vi "Log File Creater.vi"(11 "FTP log file path":path) -> (0 "all condition error":errorcluster, 2 "File Refnum":refnum<file>, 3 "Created Path":path)   [LabVIEW 2012]
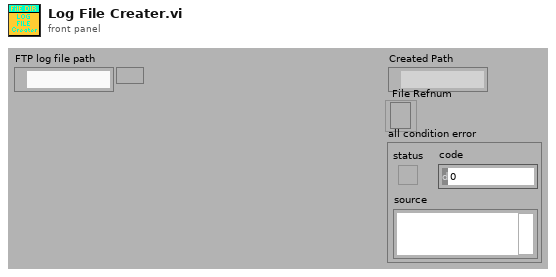
[diagram p1: front panel]
types:
  T1 = enum16{"open", "replace", "create", "open or create", "replace or create", "replace or create with confirmation"}
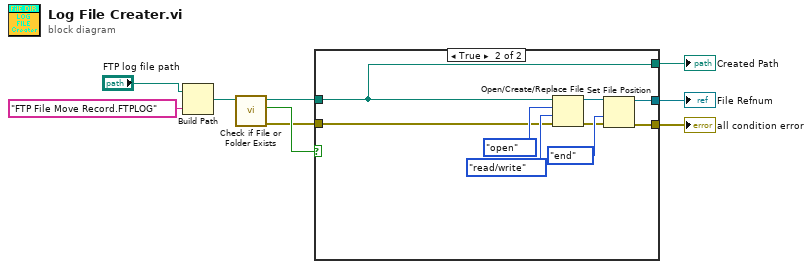
[diagram p0: block diagram]
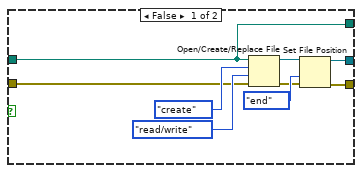
[diagram p2: hidden frame]
diagram:
  n1 = Build Path(base path="FTP log file path", name or relative path="FTP File Move Record.FTPLOG") -> (appended path=w4:path)
  n2 = call <vilib>:"Check if File or Folder Exists.vi"("path"=w4) -> ("error out"=w1:errorcluster, "file or folder exists?"=w3:bool, "dup path"=w2:path)  [unwired: 8 in]
  n3 = case shown="True" w3 {
    tunnel: [w12 w21] -> w7
    tunnel: [w11 w20] -> w9
    tunnel: [w13 w22] -> w8
    tunnel: w2 -> [w11 w20]
    tunnel: w1 -> [w10 w19]
    frame False {
      n4 = Open/Create/Replace File(file path (use dialog)=w11, error in=w10, operation (0:open)=T1."create", access (0:read/write)=enum16{"read/write", "read-only", "write-only"}."read/write") -> (refnum out=w16:refnum<file>, error out=w17:errorcluster)  [unwired: 2 in, 1 out]
      n5 = Set File Position(refnum=w16, from (0:start)=enum16{"start", "end", "current"}."end", error in=w17) -> (refnum out=w13:refnum<file>, error out=w12:errorcluster)  [unwired: 1 in]
    }
    frame True {
      n6 = Open/Create/Replace File(file path (use dialog)=w20, error in=w19, operation (0:open)=T1."open", access (0:read/write)=enum16{"read/write", "read-only", "write-only"}."read/write") -> (refnum out=w25:refnum<file>, error out=w26:errorcluster)  [unwired: 2 in, 1 out]
      n7 = Set File Position(refnum=w25, from (0:start)=enum16{"start", "end", "current"}."end", error in=w26) -> (refnum out=w22:refnum<file>, error out=w21:errorcluster)  [unwired: 1 in]
    }
  }
  "Created Path" <- w9
  "File Refnum" <- w8
  "all condition error" <- w7
